vi "Get Plot to Fit Wrapper.vi"(8 "error in (no error)":errorcluster, 11 "Fit Plot Information":T2) -> (0 "error out":errorcluster, 1 "Plot Color":u32, 2 "Plot Name":string, 3 "Plot":T1, 5 "Fit Model":T4)   [LabVIEW 2019]
uses:
  Fit Models.ctl
  Fit Plot Request Information.ctl
  <vilib>/Utility/miscctls.llb/LVPointDoubleTypeDef.ctl
  Graphs/XY Graph/XY Plot Data.ctl
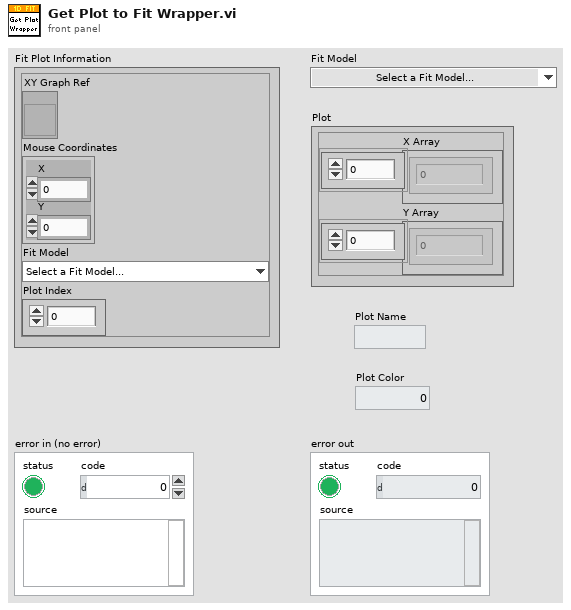
[diagram p1: front panel]
types:
  T1 = typedef "XY Plot Data.ctl" = cluster{"X Array":dbl[], "Y Array":dbl[]}
  T2 = typedef "Fit Plot Request Information.ctl" = cluster{"XY Graph Ref":refnum<vi>, "Mouse Coordinates":T3, "Fit Model":T4, "Plot Index":i32}
  T3 = typedef "LVPointDoubleTypeDef.ctl" = cluster{"X":dbl, "Y":dbl}
  T4 = typedef "Fit Models.ctl" = enum16{"Select a Fit Model...", "           Single Peak", "Gaussian", "Asymmetric Gaussian", "Lorentzian", "Asymmetric Lorentzian", "Gaussian/Lorentzian", "Lorentzian/Gaussian", "           Double Peak", "Two Gaussians", "Two Asymmetric Gaussians", "Two H-Connected Gaussians", "Two T-Connected Gaussians", "Two H-Connected Asymmetric Gaussians", "Two T-Connected Asymmetric Gaussians", "           Triple Peak", "Three Gaussians", "Three Asymmetric Gaussians", "              Decays", "1-Exponential", "IRF*PSED", "2-Exponentials", "               ACF", "2D Gaussian ACF", "2D Gaussian + Blinking ACF", "2D Gaussian + Flow ACF", "3D Gaussian ACF", "3D Gaussian + Blinking ACF", "             Multiplot", "2D Gaussian ACF & 2D Gaussian + Flow ACF"}
  T5 = typedef "XY Graph Add-Ons.lvlib/XY Graph Refnum.ctl" = refnum<vi>
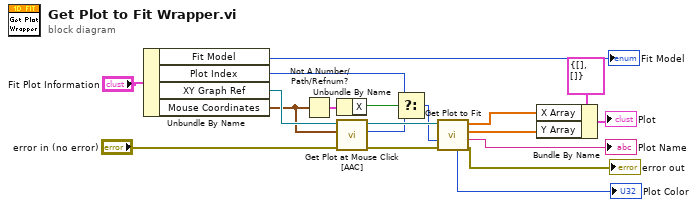
[diagram p0: block diagram]
diagram:
  n1 = Unbundle By Name("Fit Plot Information") -> ("Fit Model"=→"Fit Model":T4, "Plot Index"=w6:i32, "XY Graph Ref"=w14:refnum<vi>, "Mouse Coordinates"=w5:T3)
  n2 = Not A Number/Path/Refnum?(number/path/refnum=w5) -> (NaN/Path/Refnum?=w10:cluster{"X":bool, "Y":bool})
  n3 = Unbundle By Name(w10) -> ("X"=w9:bool)
  n4 = call "Get Plot at Mouse Click [AAC].vi"("error in (no error)"="error in (no error)", "Mouse Click Coordinates"=w5, "XYGraph Ref"=w14) -> ("error out"=w15:errorcluster, "Plot at Coordinates"=w8:i32, "XYGraph Ref"=w19:T5)  [unwired: 2 in, 4 out]
  n5 = Select(t=w6, s=w9, f=w8) -> (s? t:f=w16:i32)
  n6 = call "Get Plot to Fit.vi"("error in (no error)"=w15, "Plot Index"=w16, "XYGraph in"=w19) -> ("error out"=→"error out":errorcluster, "Plot Name"=→"Plot Name":string, "Y Array out"=w4:dbl[], "X Array out"=w3:dbl[], "Plot Color"=→"Plot Color":u32)  [unwired: 4 in]
  n7 = Bundle By Name(cluster=T1 {"X Array"=[], "Y Array"=[]} ("Plot"), "X Array"=w3, "Y Array"=w4) -> (→"Plot":T1)
